vi "Init.vi"(8 "error in (no error)":errorcluster, 11 "Profile Name":string) -> (0 "error out":errorcluster, 3 "SetCurrentProfile out":refnum<class "SetCurrentProfile.lvclass">)   [LabVIEW 2022 SP3, in "obs-websocket-lv.lvlib" / "SetCurrentProfile.lvclass"]
uses:
  SetCurrentProfile.lvclass
  SetCurrentProfile.lvclass/SetCurrentProfile.ctl
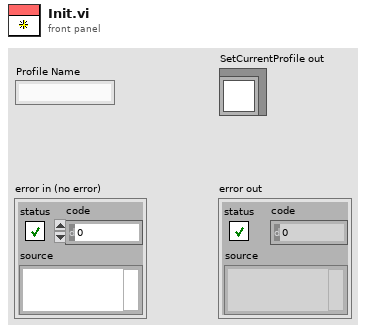
[diagram p1: front panel]
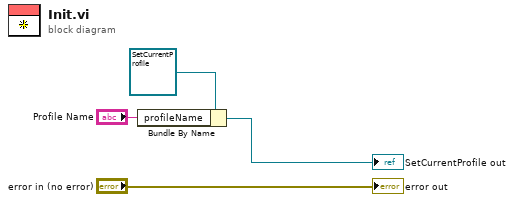
[diagram p0: block diagram]
diagram:
  n1 = Bundle By Name(cluster=refnum<class "SetCurrentProfile.lvclass"> refnum ("SetCurrentProfile in"), "profileName"="Profile Name") -> (→"SetCurrentProfile out":refnum<class "SetCurrentProfile.lvclass">)
  "error out" <- "error in (no error)"
